vi "ReadUDP.vi"() -> ()   [LabVIEW 2011]
panel:
  in  "stop":bool
  out "data out":string
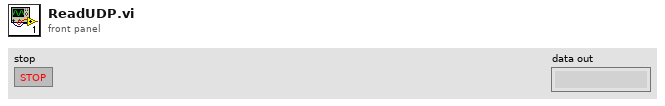
[diagram p1: front panel]
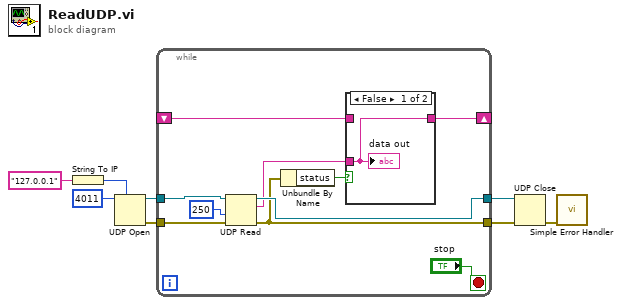
[diagram p0: block diagram]
diagram:
  n1 = String To IP(1:"127.0.0.1" ("name")) -> (0:w4:u32)
  n2 = UDP Open(7:w4, 11:u16 4011 ("port")) -> (port=w8:refnum<k16>, 0:w3:errorcluster)  [unwired: 3 in, 1 out]
  n3 = while {
    tunnel: w8 -> [w18]
    tunnel: [w17] -> w7
    shift-right: [w14] -> _
    shift-left: _ -> [w13]
    tunnel: w3 -> [w12]
    tunnel: [w11] -> w2
    stop <- "stop" stop-if-true
    n4 = UDP Read(connection ID=w18, timeout ms (25000)=250, 8:w12) -> (data out=w15:string, error out=w11:errorcluster, 3:w17:refnum<k16>)  [unwired: 1 in, 2 out]
    n5 = Unbundle By Name(w11) -> ("status"=w16:bool)
    n6 = case shown="False" w16 {
      tunnel: w15 -> [w19 _]
      tunnel: [w19 w20] -> w14
      tunnel: w13 -> [_ w20]
      frame False {
        "data out" <- w19
      }
      frame True {
      }
    }
  }
  n7 = UDP Close(connection ID=w7, 8:w2) -> (error out=w1:errorcluster)  [unwired: 1 out]
  n8 = call <vilib>:"Simple Error Handler.vi"("error in (no error)"=w1) -> ()  [unwired: 4 in, 5 out]
